vi "Motor Speed Calculation.vi"(6 "Rotation Time In":dbl format="%#.6g", 9 "Tamb":dbl format="%#_13g", 10 "Pamb":dbl format="%#_13g", 11 "Minute Volume (BTPS) In":dbl format="%#_13g") -> (2 "Minute Volume (BTPS) Out":dbl format="%#_13g", 3 "Rotation Time Out":dbl format="%#.6g")   [LabVIEW 2018]
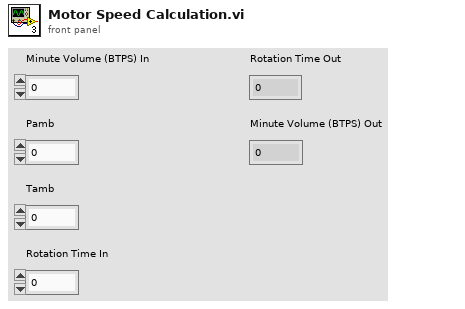
[diagram p1: front panel]
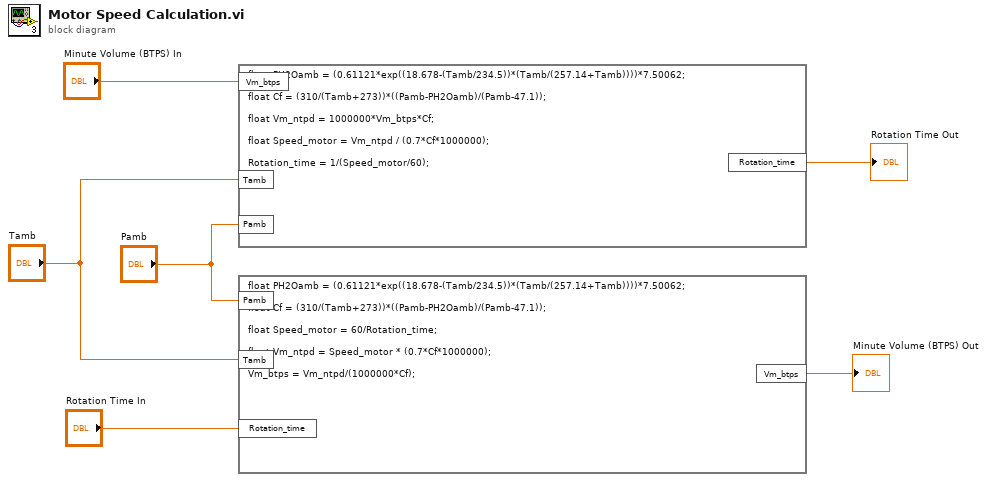
[diagram p0: block diagram]
diagram:
  n1 = formula code="float PH2Oamb = (0.61121*exp((18.678-(Tamb/234.5))*(Tamb/(257.14+Tamb))))*7.50062;\n\nfloat Cf = (310/(Tamb+273))*((Pamb-PH2Oamb)/(Pamb-47.1));\n\nfloat Vm_ntpd = 1000000*Vm_btps*Cf;\n\nfloat Speed_motor = Vm_ntpd / (0.7*Cf*1000000);\n\nRotation_time = 1/(Speed_motor/60);"("Tamb"="Tamb", "Pamb"="Pamb", "Vm_btps"="Minute Volume (BTPS) In") -> ("Rotation_time"=→"Rotation Time Out":dbl)
  n2 = formula code="float PH2Oamb = (0.61121*exp((18.678-(Tamb/234.5))*(Tamb/(257.14+Tamb))))*7.50062;\n\nfloat Cf = (310/(Tamb+273))*((Pamb-PH2Oamb)/(Pamb-47.1));\n\nfloat Speed_motor = 60/Rotation_time;\n\nfloat Vm_ntpd = Speed_motor * (0.7*Cf*1000000);\n\nVm_btps = Vm_ntpd/(1000000*Cf);"("Tamb"="Tamb", "Pamb"="Pamb", "Rotation_time"="Rotation Time In") -> ("Vm_btps"=→"Minute Volume (BTPS) Out":dbl)
